vi "Open Actor Core FP.vi"(8 "error in (no error)":errorcluster, 10 "Open FP (F)":bool, 11 "CS++BaseActor in":refnum<class "CS++BaseActor.lvclass">) -> (0 "error out":errorcluster, 3 "CS++BaseActor out":refnum<class "CS++BaseActor.lvclass">)   [LabVIEW 2013, in "CS++BaseActor.lvlib" / "CS++BaseActor.lvclass"]
doc: "Open or close <b>Actor Core.vi</B> frontpanel."
uses:
  CS++BaseActor.lvclass
  CS++BaseActor.lvclass/CS++BaseActor.ctl
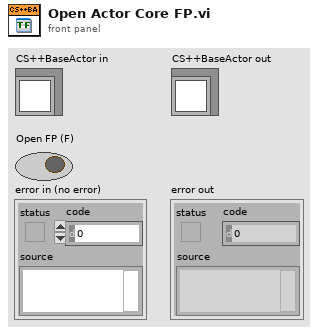
[diagram p1: front panel]
types:
  T1 = enum32{"Invalid", "Standard", "Closed", "Hidden", "Minimized", "Maximized"}
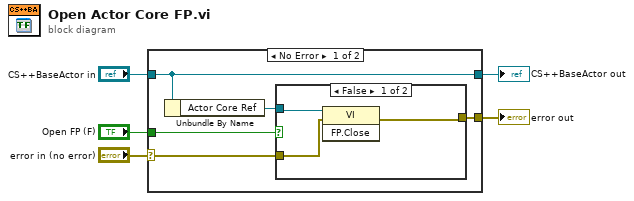
[diagram p0: block diagram]
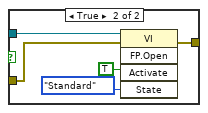
[diagram p2: hidden frame]
diagram:
  n1 = case shown="No Error" "error in (no error)" {
    selector: "error in (no error)" -> [w7 w20]
    tunnel: [w6 w20] -> w4
    tunnel: [w9 w19] -> w2
    tunnel: "CS++BaseActor in" -> [w9 w19]
    tunnel: "Open FP (F)" -> [w10 _]
    frame No Error {
      n2 = Unbundle By Name(w9) -> ("Actor Core Ref"=w8:refnum<vi>)
      n3 = case shown="False" w10 {
        tunnel: w8 -> [w13 w16]
        tunnel: w7 -> [w12 w15]
        tunnel: [w11 w14] -> w6
        frame False {
          n4 = invoke class="VI" method="FP.Close"(reference=w13, error in=w12) -> (error out=w11:errorcluster)  [unwired: 1 in, 2 out]
        }
        frame True {
          n5 = invoke class="VI" method="FP.Open"(reference=w16, error in=w15, "Activate"=TRUE ("Activate?"), "State"=T1."Standard") -> (error out=w14:errorcluster)  [unwired: 1 in, 4 out]
        }
      }
    }
    frame Error {
    }
  }
  "error out" <- w4
  "CS++BaseActor out" <- w2
